vi "GetAllAvailableRecords.vi"(8 "error in (no error)":errorcluster, 11 "Scope5761 in":refnum<class "Scope5761.lvclass">) -> (0 "error out":errorcluster, 2 "Available records":i32, 3 "Scope5761 out":refnum<class "Scope5761.lvclass">)   [LabVIEW 2013, in "Scope5761.lvclass"]
uses:
  Scope5761.lvclass
  Scope5761.lvclass/Scope5761.ctl
  FpgaRef/FpgaRef5761/FpgaRef5761.lvclass
  FpgaRef/FpgaRef5782/FpgaRef5782.lvclass
  FpgaRef/FpgaRefBase/FpgaRefBase.lvclass
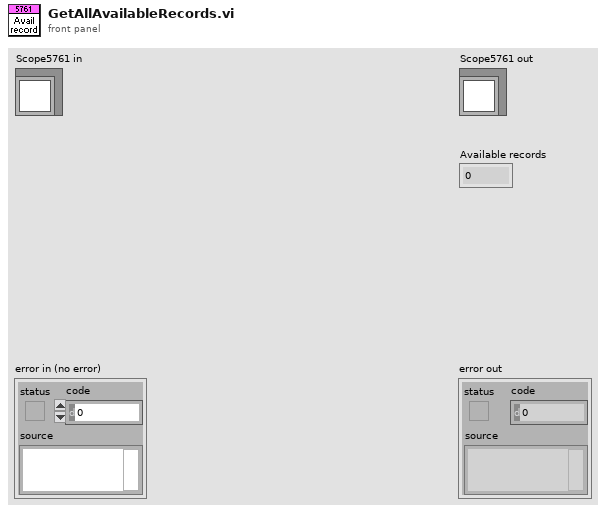
[diagram p1: front panel]
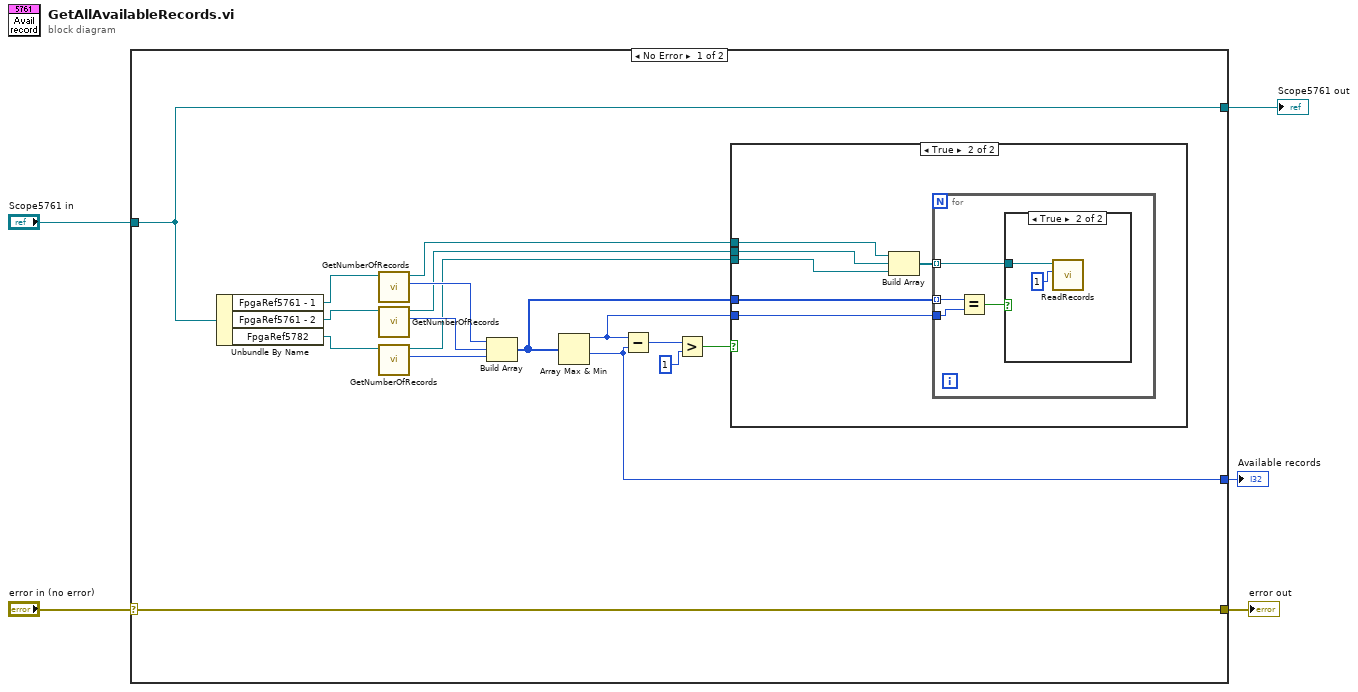
[diagram p0: block diagram]
diagram:
  n1 = case shown="No Error" "error in (no error)" {
    selector: "error in (no error)" -> [w22 w36]
    tunnel: [w22 w36] -> w4
    tunnel: [w6 w35] -> w2
    tunnel: "Scope5761 in" -> [w6 w35]
    tunnel: [w10 _] -> w1
    frame No Error {
      n2 = Unbundle By Name(w6) -> ("FpgaRef5761 - 1"=w21:refnum<class "FpgaRef5761.lvclass">, "FpgaRef5761 - 2"=w20:refnum<class "FpgaRef5761.lvclass">, "FpgaRef5782"=w19:refnum<class "FpgaRef5782.lvclass">)
      n3 = call-dynamic "GetNumberOfRecords.vi"("FpgaRef5761 In"=w21) -> ("number of records"=w18:i32, "FpgaRef5761 Out"=w9:refnum<class "FpgaRef5761.lvclass">)  [unwired: 8 in, 1 out]
      n4 = call-dynamic "GetNumberOfRecords.vi"("FpgaRef5761 In"=w20) -> ("number of records"=w17:i32, "FpgaRef5761 Out"=w8:refnum<class "FpgaRef5761.lvclass">)  [unwired: 8 in, 1 out]
      n5 = call-dynamic "GetNumberOfRecords.vi"("FpgaRef5782 in"=w19) -> ("number of records"=w16:i32, "FpgaRef5782 out"=w7:refnum<class "FpgaRef5782.lvclass">)  [unwired: 8 in, 1 out]
      n6 = Build Array(w18, w17, w16) -> (w12:i32[])
      n7 = Array Max & Min(array=w12) -> (max value=w11:i32, min value=w10:i32)  [unwired: 2 out]
      n8 = Subtract(x=w11, y=w10) -> (x-y=w15:i32)
      n9 = Greater?(x=w15, y=1) -> (0:w13:bool)
      n10 = case shown="True" w13 {
        tunnel: w12 -> [_ w27]
        tunnel: w11 -> [_ w26]
        tunnel: w9 -> [_ w25]
        tunnel: w8 -> [_ w24]
        tunnel: w7 -> [_ w23]
        frame False {
        }
        frame True {
          n11 = Build Array(w25, w24, w23) -> (w28:refnum<class "FpgaRefBase.lvclass">[])
          n12 = for {
            tunnel: w28 -> [w30] mode=indexing
            tunnel: w27 -> [w32] mode=indexing
            tunnel: w26 -> [w31]
            n13 = Equal?(x=w32, y=w31) -> (x = y?=w29:bool)
            n14 = case shown="True" w29 {
              tunnel: w30 -> [_ w34]
              frame False {
              }
              frame True {
                n15 = call-dynamic "ReadRecords.vi"("Num records to read"=1, "FpgaRefBase in"=w34) -> ()  [unwired: 7 in, 3 out]
              }
            }
          }
        }
      }
    }
    frame Error {
    }
  }
  "error out" <- w4
  "Scope5761 out" <- w2
  "Available records" <- w1
